vi "Write_summary_file.vi"(5 "Dust Array":T1[](array[typedef]) {"File Location" items=["Currently Writing"=-3, "Labview Files"=-2, "Mars Data Processing Factility"=-1, "Local Cache "=0, "Old Storage"=1, "Storage"=2]; "Estimate Source" items=["Any Source."=-2, "No Shot"=-1, "Basic Labview Estimate"=0, "IDL Estimate From Andrew"=1, "IDL Estimate From Tobin"=2, "Old Metadata"=3]}, 8 "error in (no error)":errorcluster, 11 "ref":i32) -> (0 "error out":errorcluster, 3 "ref out":i32)   [LabVIEW 2012]
uses:
  Public API/Query_Dust_Event.ctl
  Estimate_source.ctl
  File_location.ctl
  <vilib>/addons/h5labview/H5GroupObject.lvlib
panel:
  # "Dust Event"
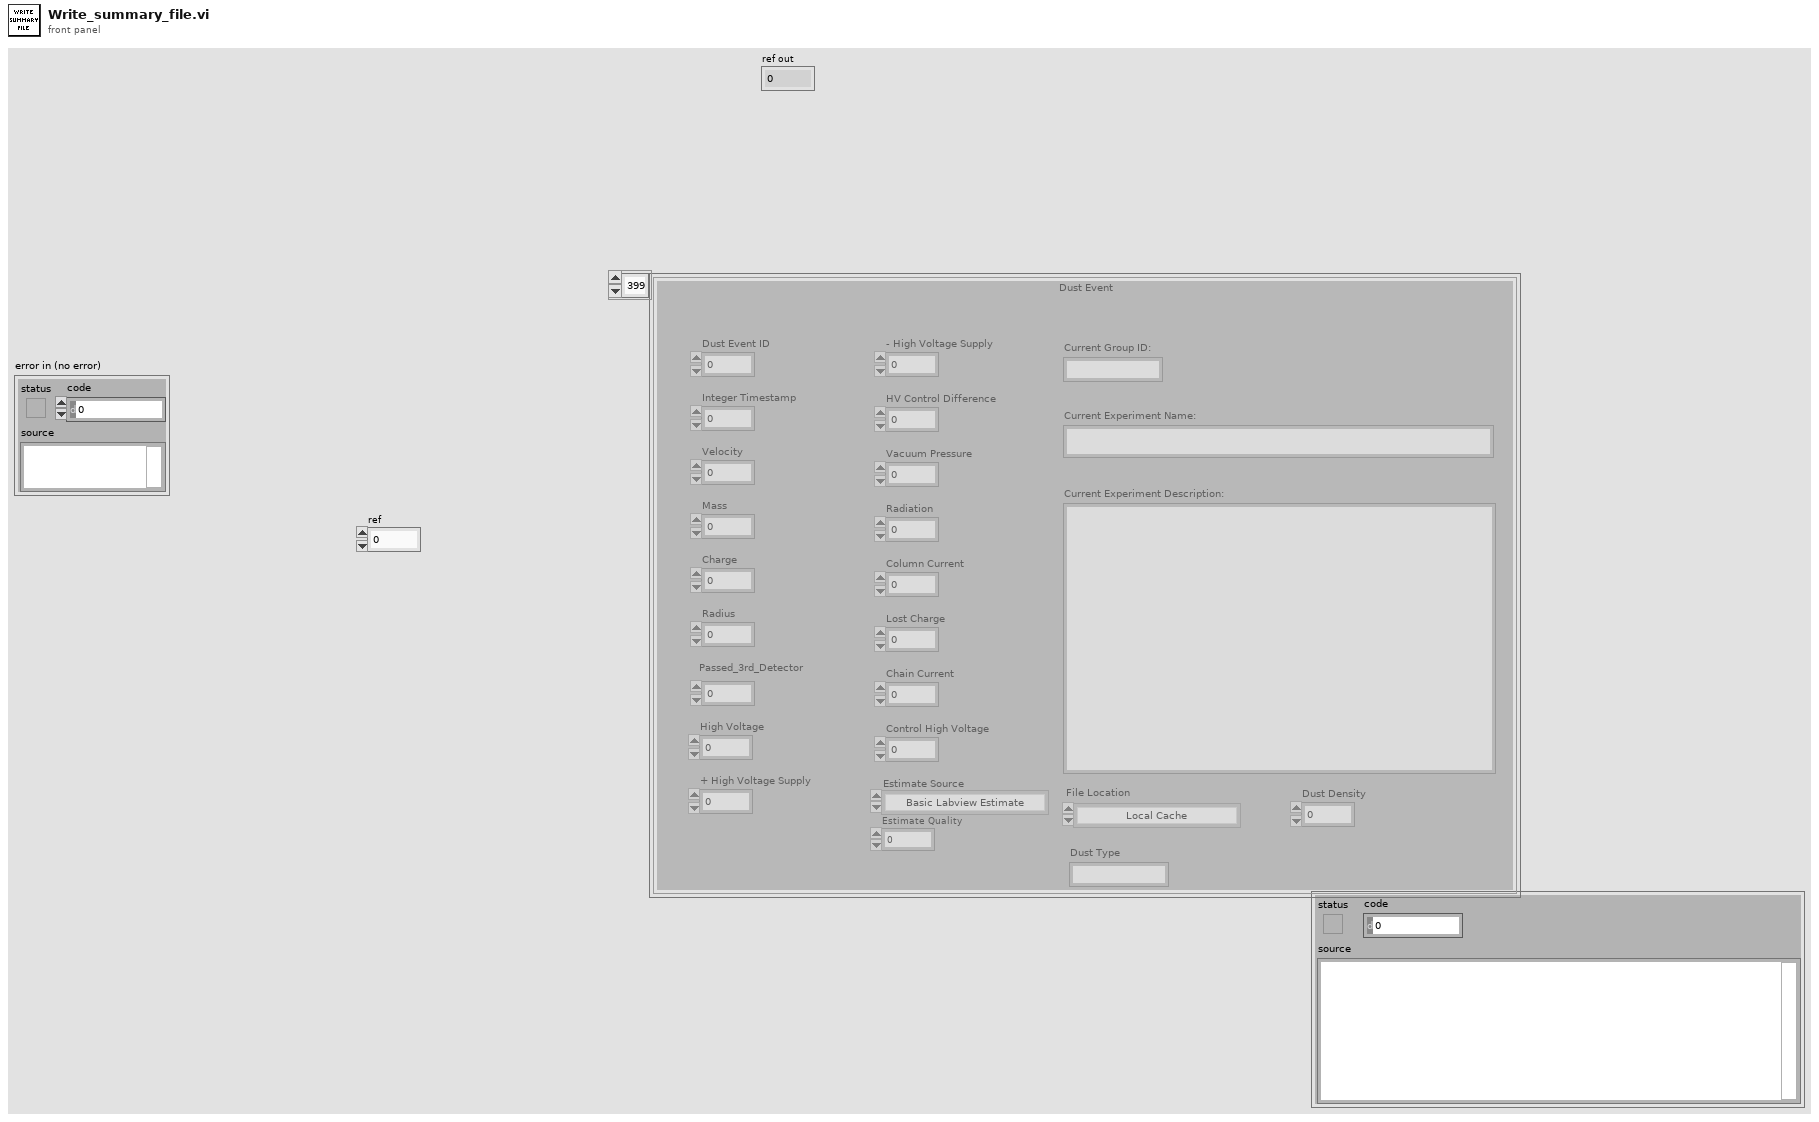
[diagram p1: front panel]
types:
  T1 = typedef "Query_Dust_Event.ctl" = cluster{"Dust Event ID":i64, "Integer Timestamp":i64, "Velocity":sgl, "Mass":sgl, "Charge":sgl, "Radius":sgl, "Passed_3rd_Detector":i8, "High Voltage":sgl, "+ High Voltage Supply":sgl, "- High Voltage Supply":sgl, "HV Control Difference":sgl, "Vacuum Pressure":sgl, "Radiation":sgl, "Column Current":sgl, "Lost Charge":sgl, "Chain Current":sgl, "Control High Voltage":sgl, "Current Group ID:":string, "Current Experiment Name:":string, "Current Experiment Description:":string, "Estimate Source":T2, "Estimate Quality":sgl, "File Location":T3, "Dust Type":string, "Dust Density":sgl}
  T2 = typedef "Estimate_source.ctl" = i8
  T3 = typedef "File_location.ctl" = i8
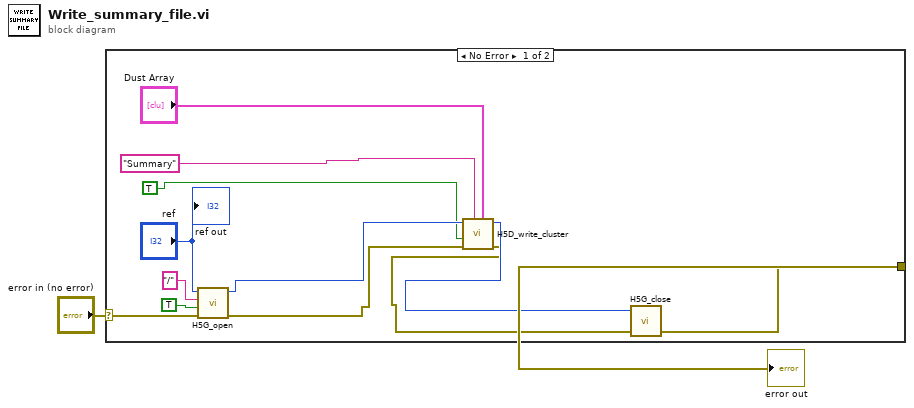
[diagram p0: block diagram]
diagram:
  n1 = case shown="No Error" "error in (no error)" {
    selector: "error in (no error)" -> [w12 w15]
    tunnel: [w10 w15] -> w1
    frame No Error {
      n2 = call <vilib>:"H5G_open.vi"("error in (no error)"=w12, "create? (F)"=TRUE, "name"="/", "ref"="ref") -> ("error out"=w4:errorcluster, "group"=w7:i32)  [unwired: 2 in]
      n3 = call "H5D_write_cluster.vi"("Dust Array"="Dust Array", "name"="Summary", "error in (no error)"=w4, "overwrite?"=TRUE, "ref"=w7) -> ("error out"=w5:errorcluster, "ref out"=w6:i32)  [unwired: 3 in]
      n4 = call <vilib>:"H5G_close.vi"("error in (no error)"=w5, "ref"=w6) -> ("error out"=w10:errorcluster)  [unwired: 3 in]
      "ref out" <- "ref"
    }
    frame Error {
    }
  }
  "error out" <- w1
